vi "CRYDB Insert Into CurveTable .vi"(8 "error in":errorcluster, 10 "Curve_Table Data":T1, 11 "connection reference":T2) -> (0 "error out":errorcluster, 2 "Curve ID":i32, 3 "connection reference out":T2)   [LabVIEW 2013]
uses:
  <vilib>/addons/database/Connection.llb/Conn ObjectReference.ctl
  <vilib>/addons/database/Auxilliary.llb/DB Tools Column Info.ctl
  <vilib>/addons/database/Auxilliary.llb/DB Tools DataTypes.ctl
  <vilib>/addons/database/Connection.llb/Conn Execute.vi
  <vilib>/addons/database/Recordset.llb/Rec Fetch Recordset Data (R).vi
  <vilib>/addons/database/Recordset.llb/Rec Destroy - Connection.vi
  <vilib>/addons/database/_DB Variant To Data/Database Variant To Data.xnode
  <vilib>/addons/database/NI_Database_API.lvlib
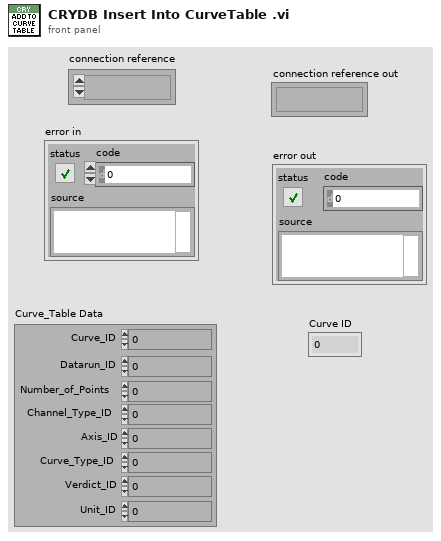
[diagram p1: front panel]
types:
  T1 = cluster{"Curve_ID":u32, "Datarun_ID":i32, "Number_of_Points":i32, "Channel_Type_ID":i32, "Axis_ID":i32, "Curve_Type_ID":i32, "Verdict_ID":i32, "Unit_ID":i32}
  T2 = typedef "NI_Database_API.lvlib/Conn ObjectReference.ctl" = refnum<k1>
  T3 = typedef "NI_Database_API.lvlib/DB Tools Column Info.ctl" = cluster{"column name":string, "data type":T4, "size":i32, "allow null?":bool}
  T4 = typedef "NI_Database_API.lvlib/DB Tools DataTypes.ctl" = enum16{"String", "Long (I32)", "Single (SGL)", "Double (DBL)", "Date/Time", "Binary"}
  T5 = typedef "NI_Database_API.lvlib/Rec ObjectReference.ctl" = refnum<k1>
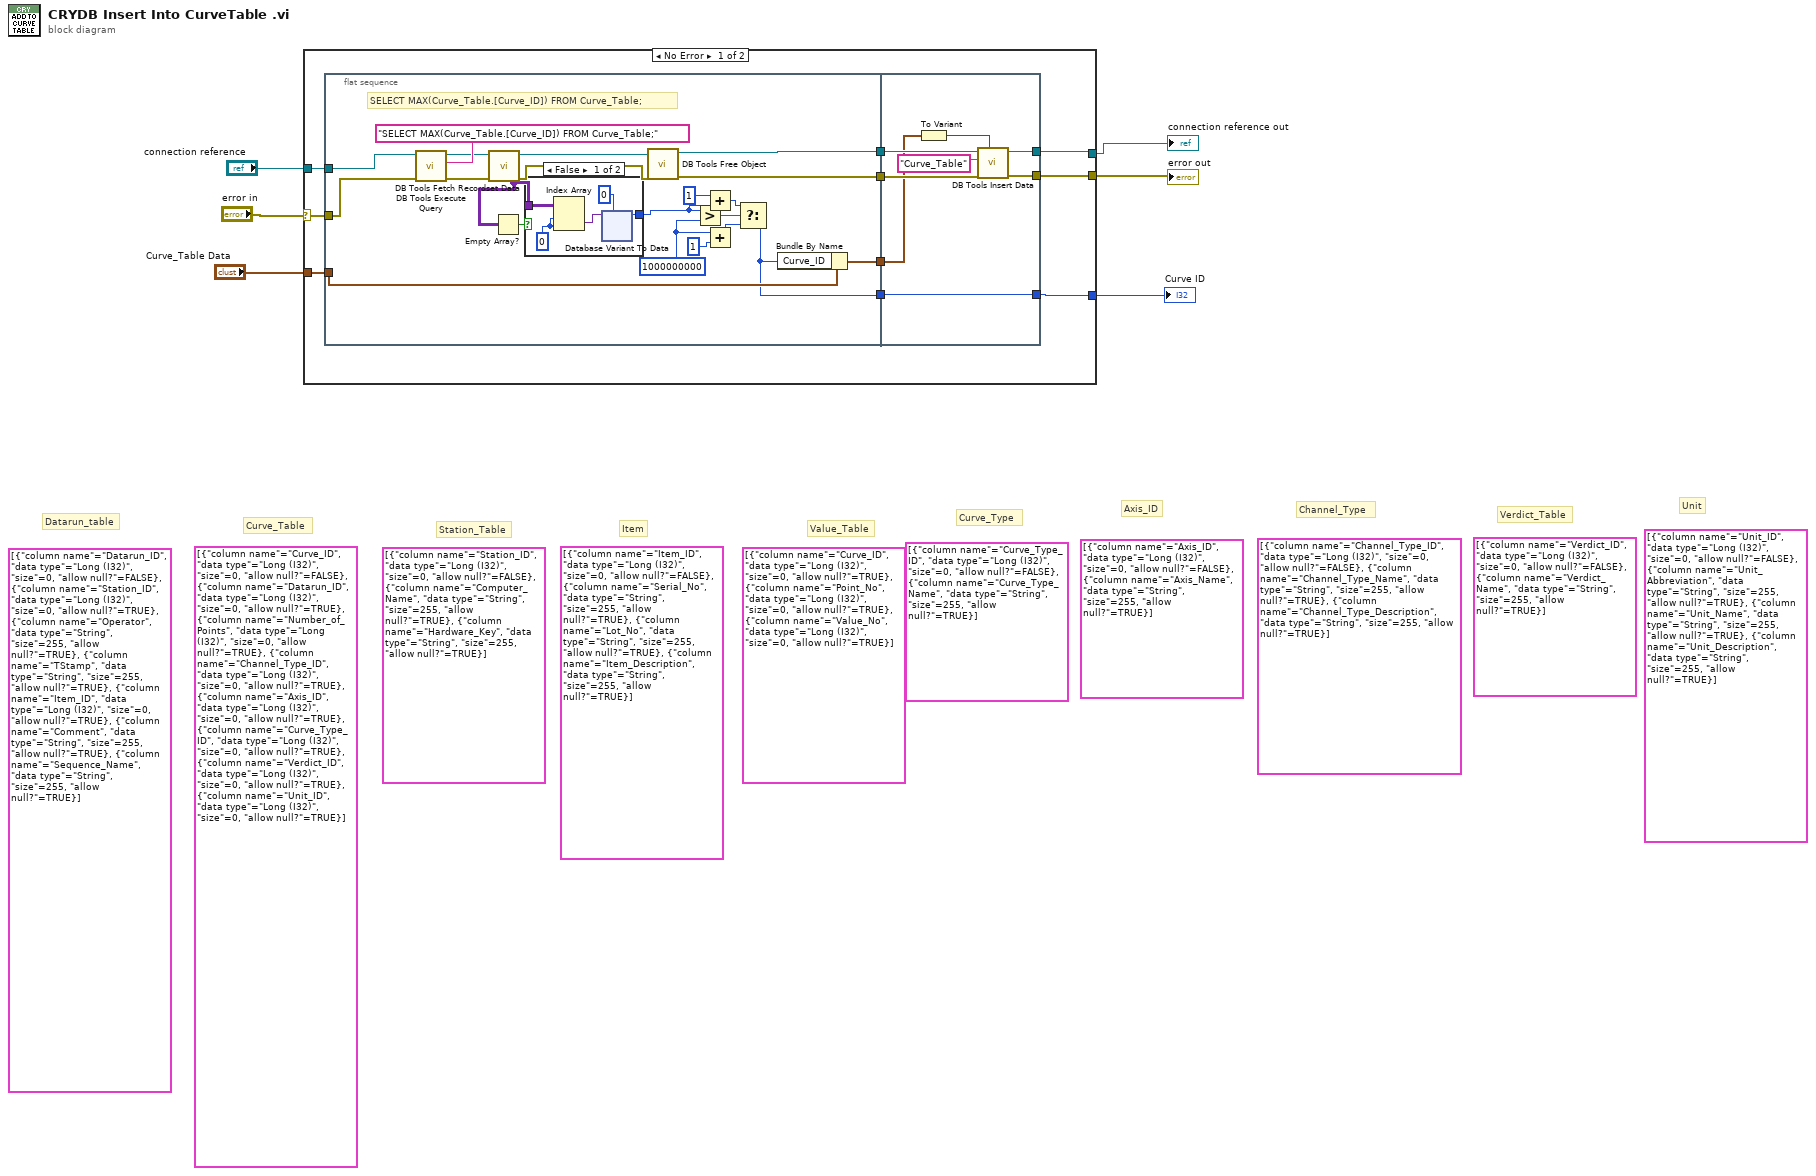
[diagram p0: block diagram]
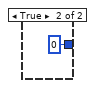
[diagram p2: hidden frame]
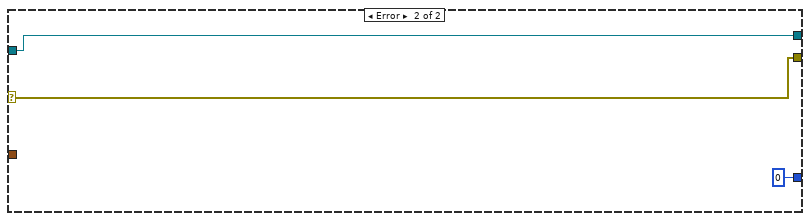
[diagram p3: hidden frame]
diagram:
  (unwired) T3[] [{"column name"="Unit_ID", "data type"=enum."Long (I32)", "size"=0, "allow null?"=FALSE}, {"column name"="Unit_Abbreviation", "data type"=enum."String", "size"=255, "allow null?"=TRUE}, {"column name"="Unit_Name", "data type"=enum."String", "size"=255, "allow null?"=TRUE}, {"column name"="Unit_Description", "data type"=enum."String", "size"=255, "allow null?"=TRUE}] ("column information")
  (unwired) T3[] [{"column name"="Verdict_ID", "data type"=enum."Long (I32)", "size"=0, "allow null?"=FALSE}, {"column name"="Verdict_Name", "data type"=enum."String", "size"=255, "allow null?"=TRUE}] ("column information")
  (unwired) T3[] [{"column name"="Channel_Type_ID", "data type"=enum."Long (I32)", "size"=0, "allow null?"=FALSE}, {"column name"="Channel_Type_Name", "data type"=enum."String", "size"=255, "allow null?"=TRUE}, {"column name"="Channel_Type_Description", "data type"=enum."String", "size"=255, "allow null?"=TRUE}] ("column information")
  (unwired) T3[] [{"column name"="Axis_ID", "data type"=enum."Long (I32)", "size"=0, "allow null?"=FALSE}, {"column name"="Axis_Name", "data type"=enum."String", "size"=255, "allow null?"=TRUE}] ("column information")
  (unwired) T3[] [{"column name"="Curve_Type_ID", "data type"=enum."Long (I32)", "size"=0, "allow null?"=FALSE}, {"column name"="Curve_Type_Name", "data type"=enum."String", "size"=255, "allow null?"=TRUE}] ("column information")
  (unwired) T3[] [{"column name"="Curve_ID", "data type"=enum."Long (I32)", "size"=0, "allow null?"=TRUE}, {"column name"="Point_No", "data type"=enum."Long (I32)", "size"=0, "allow null?"=TRUE}, {"column name"="Value_No", "data type"=enum."Long (I32)", "size"=0, "allow null?"=TRUE}] ("column information")
  (unwired) T3[] [{"column name"="Item_ID", "data type"=enum."Long (I32)", "size"=0, "allow null?"=FALSE}, {"column name"="Serial_No", "data type"=enum."String", "size"=255, "allow null?"=TRUE}, {"column name"="Lot_No", "data type"=enum."String", "size"=255, "allow null?"=TRUE}, {"column name"="Item_Description", "data type"=enum."String", "size"=255, "allow null?"=TRUE}] ("column information")
  (unwired) T3[] [{"column name"="Station_ID", "data type"=enum."Long (I32)", "size"=0, "allow null?"=FALSE}, {"column name"="Computer_Name", "data type"=enum."String", "size"=255, "allow null?"=TRUE}, {"column name"="Hardware_Key", "data type"=enum."String", "size"=255, "allow null?"=TRUE}] ("column information")
  (unwired) T3[] [{"column name"="Curve_ID", "data type"=enum."Long (I32)", "size"=0, "allow null?"=FALSE}, {"column name"="Datarun_ID", "data type"=enum."Long (I32)", "size"=0, "allow null?"=TRUE}, {"column name"="Number_of_Points", "data type"=enum."Long (I32)", "size"=0, "allow null?"=TRUE}, {"column name"="Channel_Type_ID", "data type"=enum."Long (I32)", "size"=0, "allow null?"=TRUE}, {"column name"="Axis_ID", "data type"=enum."Long (I32)", "size"=0, "allow null?"=TRUE}, {"column name"="Curve_Type_ID", "data type"=enum."Long (I32)", "size"=0, "allow null?"=TRUE}, {"column name"="Verdict_ID", "data type"=enum."Long (I32)", "size"=0, "allow null?"=TRUE}, {"column name"="Unit_ID", "data type"=enum."Long (I32)", "size"=0, "allow null?"=TRUE}] ("column information")
  (unwired) T3[] [{"column name"="Datarun_ID", "data type"=enum."Long (I32)", "size"=0, "allow null?"=FALSE}, {"column name"="Station_ID", "data type"=enum."Long (I32)", "size"=0, "allow null?"=TRUE}, {"column name"="Operator", "data type"=enum."String", "size"=255, "allow null?"=TRUE}, {"column name"="TStamp", "data type"=enum."String", "size"=255, "allow null?"=TRUE}, {"column name"="Item_ID", "data type"=enum."Long (I32)", "size"=0, "allow null?"=TRUE}, {"column name"="Comment", "data type"=enum."String", "size"=255, "allow null?"=TRUE}, {"column name"="Sequence_Name", "data type"=enum."String", "size"=255, "allow null?"=TRUE}] ("column information")
  # "Unit"
  # "Verdict_Table"
  # "Channel_Type"
  # "Axis_ID"
  # "Curve_Type"
  # "Value_Table"
  # "Item"
  # "Station_Table"
  # "Curve_Table"
  # "Datarun_table"
  n1 = case shown="No Error" "error in" {
    selector: "error in" -> [w12 w85]
    tunnel: "connection reference" -> [w16 w86]
    tunnel: "Curve_Table Data" -> [w15 _]
    tunnel: [w10 w86] -> w2
    tunnel: [w9 w85] -> w3
    tunnel: [w7 0] -> w1
    frame No Error {
      n2 = flat-sequence {
        tunnel: w16 -> [w37]
        tunnel: w15 -> [w32]
        tunnel: [w33] -> w14
        tunnel: [w25] -> w13
        tunnel: w12 -> [w24]
        tunnel: [w21] -> w11
        tunnel: [w20] -> w8
        tunnel: w14 -> [w83]
        tunnel: w13 -> [w77]
        tunnel: w11 -> [w81]
        tunnel: [w79] -> w10
        tunnel: [w78] -> w9
        tunnel: w8 -> [w76]
        tunnel: [w76] -> w7
        frame #0 {
          w28 = 1000000000 ("y")
          # "SELECT MAX(Curve_Table.[Curve_ID]) FROM Curve_Table;"
          n3 = call-poly <vilib>:"DB Tools Execute Query.vi"("error in (no error)"=w24, "SQL query"="SELECT MAX(Curve_Table.[Curve_ID]) FROM Curve_Table;", "connection reference"=w37) -> ("error out"=w23:errorcluster, "recordset reference"=w35:T5)  [unwired: 5 in]
          n4 = call-poly <vilib>:"DB Tools Fetch Recordset Data.vi"("error in (no error)"=w23, "recordset reference"=w35) -> ("error out"=w22:errorcluster, "recordset data"=w17:variant[][], "recordset reference out"=w34:T5)  [unwired: 3 in]
          n5 = Empty Array?(array=w17) -> (empty?=w19:bool)
          n6 = case shown="False" w19 {
            tunnel: w17 -> [w42 _]
            tunnel: [w39 0 ("data")] -> w18
            frame False {
              w41 = 0 ("disabled index (col)")
              n7 = Index Array(array=w42, index (row)=w41, index (col)=w41) -> (element=w38:variant)
              n8 = xnode "Database Variant To Data"("database variant"=w38, "type"=0) -> ("data"=w39:i32)  [unwired: 1 in, 1 out]
            }
            frame True {
            }
          }
          n9 = call-poly <vilib>:"DB Tools Free Object.vi"("error in (no error)"=w22, "recordset reference"=w34) -> ("error out"=w21:errorcluster, "connection reference"=w33:T2)  [unwired: 8 in]
          n10 = Greater?(x=w18, y=w28) -> (0:w31:bool)
          n11 = Add(x=1, y=w18) -> (x+y=w26:i32)
          n12 = Add(x=w28, y=1 ("x")) -> (x+y=w29:i32)
          n13 = Select(t=w26, s=w31, f=w29) -> (s? t:f=w20:i32)
          n14 = Bundle By Name(cluster=w32, "Curve_ID"=w20) -> (w25:T1)
        }
        frame #1 {
          n15 = To Variant(anything=w77) -> (Variant=w80:variant)
          n16 = call <vilib>:"DB Tools Insert Data.vi"("data"=w80, "error in (no error)"=w81, "table"="Curve_Table", "connection reference"=w83) -> ("error out"=w78:errorcluster, "connection reference out"=w79:T2)  [unwired: 6 in]
        }
      }
    }
    frame Error {
    }
  }
  "connection reference out" <- w2
  "error out" <- w3
  "Curve ID" <- w1
